vi "ReadDataFileHDF5PMT.vi"(8 "error in (no error) 2":errorcluster, 10 "File Paths":T1={"Local Save Path"=path "\\\\smbhome.uscs.susx.ac.uk\\cv222/Desktop/data", "Newton Save Path"=path "Z:/#Projects/Entanglement/data", "File Name"="test", "LocalSave"=TRUE}, 11 "step":i32) -> (0 "error out 2":errorcluster, 3 "last step data":i32[][](array[numeric]))   [LabVIEW 2019]
uses:
  controls/FilePaths.ctl
  <vilib>/UPVI/lvhdf5/file.llb/LVH5F Operation.ctl
  controls/GlobalExp.vi
  <vilib>/UPVI/lvhdf5/dataset.llb/H5Dread (Variant).vi
  <vilib>/UPVI/lvhdf5/library.llb/HDF5 Ref.ctl
  <vilib>/UPVI/lvhdf5/dataset.llb/H5Dread.xnode
  Global.lvlib
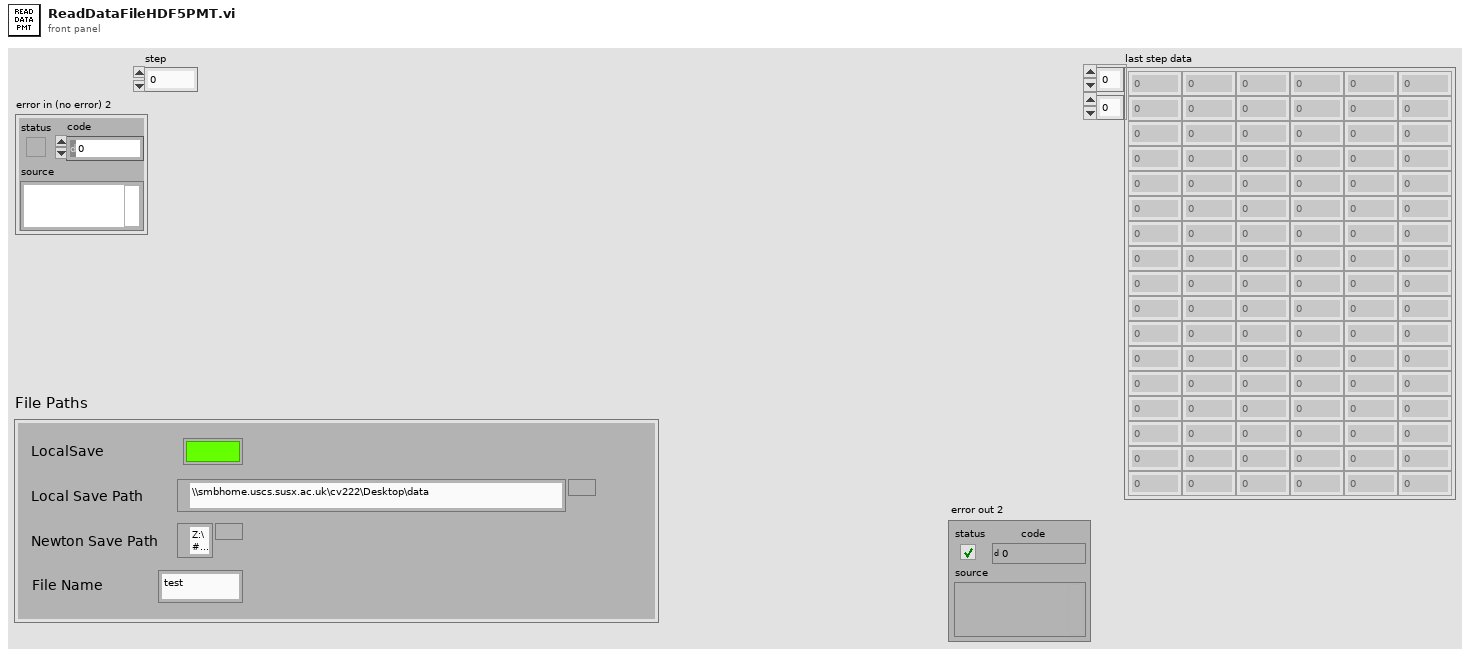
[diagram p1: front panel]
types:
  T1 = typedef "FilePaths.ctl" = cluster{"Local Save Path":path, "Newton Save Path":path, "File Name":string, "LocalSave":bool}
  T2 = typedef "LVH5F Operation.ctl" = enum16{"open", "open or create", "create or replace", "create or replace (with confirmation)", "create", "open (read only)"}
  T3 = typedef "MasterExpControl.ctl" = cluster{"Main Steps":dbl, "Main Runs":dbl, "ExpStatus":enum16{"Innit", "Stop", "Idle", "MainRunning", "AuxRunning"}, "Main Current Step":dbl, "ExpNum":dbl, "NewData":bool, "date":string, "command":string, "Stop":bool, "Pause":bool, "Mathematica":string, "Main/Meta":bool, "UpdateMath":bool, "Camera":bool, "MetaExpOver":bool, "NextMetaExp":bool}
  T4 = typedef "HDF5 Ref.ctl" = refnum<k1>
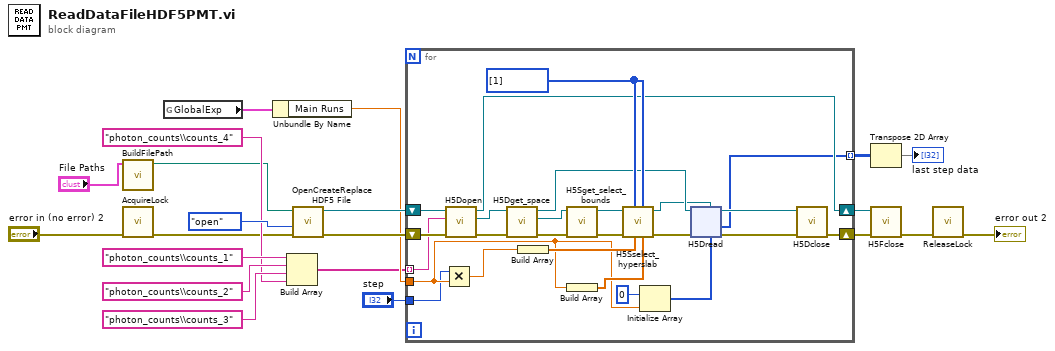
[diagram p0: block diagram]
diagram:
  n1 = call "BuildFilePath.vi"("File Paths"="File Paths") -> ("appended path"=w1:path)  [unwired: 10 in]
  n2 = call "AcquireLock.vi"("error in (no error)"="error in (no error) 2") -> ("error out"=w5:errorcluster)  [unwired: 10 in]
  n3 = global read "GlobalExp.vi" "GlobalExp"() -> (w21:T3)
  n4 = Unbundle By Name(w21) -> ("Main Runs"=w15:dbl)
  n5 = Build Array("photon_counts\\counts_1" ("Dataset Path"), "photon_counts\\counts_2" ("Dataset Path"), "photon_counts\\counts_3" ("Dataset Path"), "photon_counts\\counts_4" ("Dataset Path")) -> (w10:string[])
  n6 = call <vilib>:"OpenCreateReplace HDF5 File.vi"("error in (no error)"=w5, "function (open or create)"=LVH5F_Operation."open", "path"=w1) -> ("error out"=w18:errorcluster, "HDF5 Ref out"=w19:T4)  [unwired: 5 in]
  n7 = for {
    tunnel: w15 -> [w25]
    shift-right: [w27] -> w16
    shift-left: w19 -> [w46]
    shift-right: [w28] -> w17
    shift-left: w18 -> [w45]
    tunnel: w10 -> [w26] mode=indexing
    tunnel: [w22] -> w9 mode=indexing
    tunnel: "step" -> [w24]
    w42 = u64[] [1] ("Stride")
    n8 = Multiply(x=w24, y=w25) -> (x*y=w23:dbl)
    n9 = call <vilib>:"H5Dopen.vi"("error in (no error)"=w45, "name"=w26, "HDF5 Ref"=w46) -> ("error out"=w43:errorcluster, "HDF5 Dataset Ref"=w44:T4, "HDF5 Ref out"=w27:T4)  [unwired: 4 in]
    n10 = call <vilib>:"H5Dget_space.vi"("error in (no error)"=w43, "HDF5 Dataset Ref"=w44) -> ("error out"=w37:errorcluster, "HDF5 Dataspace Ref"=w39:T4, "HDF5 Dataset Ref out"=w35:T4)  [unwired: 5 in]
    n11 = Build Array(w23) -> (w40:dbl[])
    n12 = call <vilib>:"H5Sget_select_bounds.vi"("error in (no error)"=w37, "HDF5 Space Ref"=w39) -> ("error out"=w36:errorcluster, "HDF5 Ref out"=w38:T4)  [unwired: 4 in, 2 out]
    n13 = Build Array(w25) -> (w41:dbl[])
    n14 = call <vilib>:"H5Sselect_hyperslab.vi"("Count"=w41, "Block"=w42, "Start"=w40, "Stride"=w42, "error in (no error)"=w36, "HDF5 Space Ref"=w38) -> ("error out"=w34:errorcluster, "HDF5 Ref out"=w31:T4)  [unwired: 4 in]
    n15 = Initialize Array(u64 0, w25) -> (w32:u64[])
    n16 = xnode "H5Dread"("HDF5 Dataset Ref"=w35, "HDF5 File Space (H5S_ALL)"=w31, "error in (no error)"=w34, "Data"=w32) -> ("HDF5 Dataset Ref out"=w29:T4, "error out"=w30:errorcluster, "Data out"=w22:u64[])  [unwired: 3 in]
    n17 = call <vilib>:"H5Dclose.vi"("error in (no error)"=w30, "HDF5 Dataset Ref"=w29) -> ("error out"=w28:errorcluster)  [unwired: 7 in]
  }
  n18 = Transpose 2D Array(2D array=w9) -> (transposed array=→"last step data":u64[][])
  n19 = call <vilib>:"H5Fclose.vi"("error in (no error)"=w17, "HDF5 Ref"=w16) -> ("error out"=w4:errorcluster)  [unwired: 7 in]
  n20 = call "ReleaseLock.vi"("error in (no error)"=w4) -> ("error out"=→"error out 2":errorcluster)  [unwired: 10 in]
